vi "BBO_Spare.vi"(9 "카메라 X":dbl=12.0, 11 "클러스터":T2={{"정지할 차이값"=0.08, "흰색과 밖 차이값"=0.15, "흰/검 반 값 "=0.3}, {"4: 오른각도"=122.0, "4: 뒷쪽각도"=0.0, "5: 오른각도"=120.0, "5: 앞쪽각도"=245.0, "6: 왼쪽각도"=245.0, "6: 앞쪽각도"=120.0}, {"2: 공각도"=233.0, "2: 굴릴각도"=60.0}}) -> (3 "ROI":T1={"Global Rectangle"=[536, 448, 795, 574], "Contours"=[{"Contour Type"=0, "ROI Type"=3, "Points"=[536, 448, 795, 574]}]})   [LabVIEW 2014]
doc: "The myRIO Project template acquires acceleration data from the onboard accelerometer and displays the changes of acceleration values in a waveform chart."
uses:
  <vilib>/userdefined/High Color/IMAQdx.ctl
  <vilib>/vision/driver/NI_Vision_Acquisition_Software.lvlib
  <vilib>/vision/NI_Vision_Development_Module.lvlib
panel:
  out "시간체크":u32=8202
  in  "Range":cluster{"Lower value":sgl, "Upper value":sgl}={"Lower value"=128.0, "Upper value"=255.0} {"Upper value" format="%.2f"; "Lower value" format="%.2f"}
  in  "조정":dbl=300.0
  in  "수평(뒤로) 초":u32=150
  out "Number of Particles":i32=4
  in  "Local":T3={"Object Type"=0, "Method"=1, "Niblack Deviation Factor"=1.0, "Window"={"Width"=20, "Height"=20}} {"Niblack Deviation Factor" min=0.0 max=1.0 format="%.2f"; "Method" items=["Niblack", "Background Correction"]; "Object Type" items=["Bright Objects", "Dark Objects"]}
  out "숫자형 컨트롤":i32=8
  in  "Select Servo 2":string(combo)="Servo 2"
  out "볼링핀을찾았는가":bool=TRUE
  in  "공 굴릴 범위":dbl=5.0
  in  "작게 움직이는 범위":dbl=500.0
  in  "좌우모터":i16=25
  out "Image 2":T4(plugin-control)
  out "Image":T4(plugin-control)
  # "Control Motor"
  # "Read Encoder"
  # "중간 22"
  # "25"
  # "1,3핀 12"
  # "1일때 + 0일때 -"
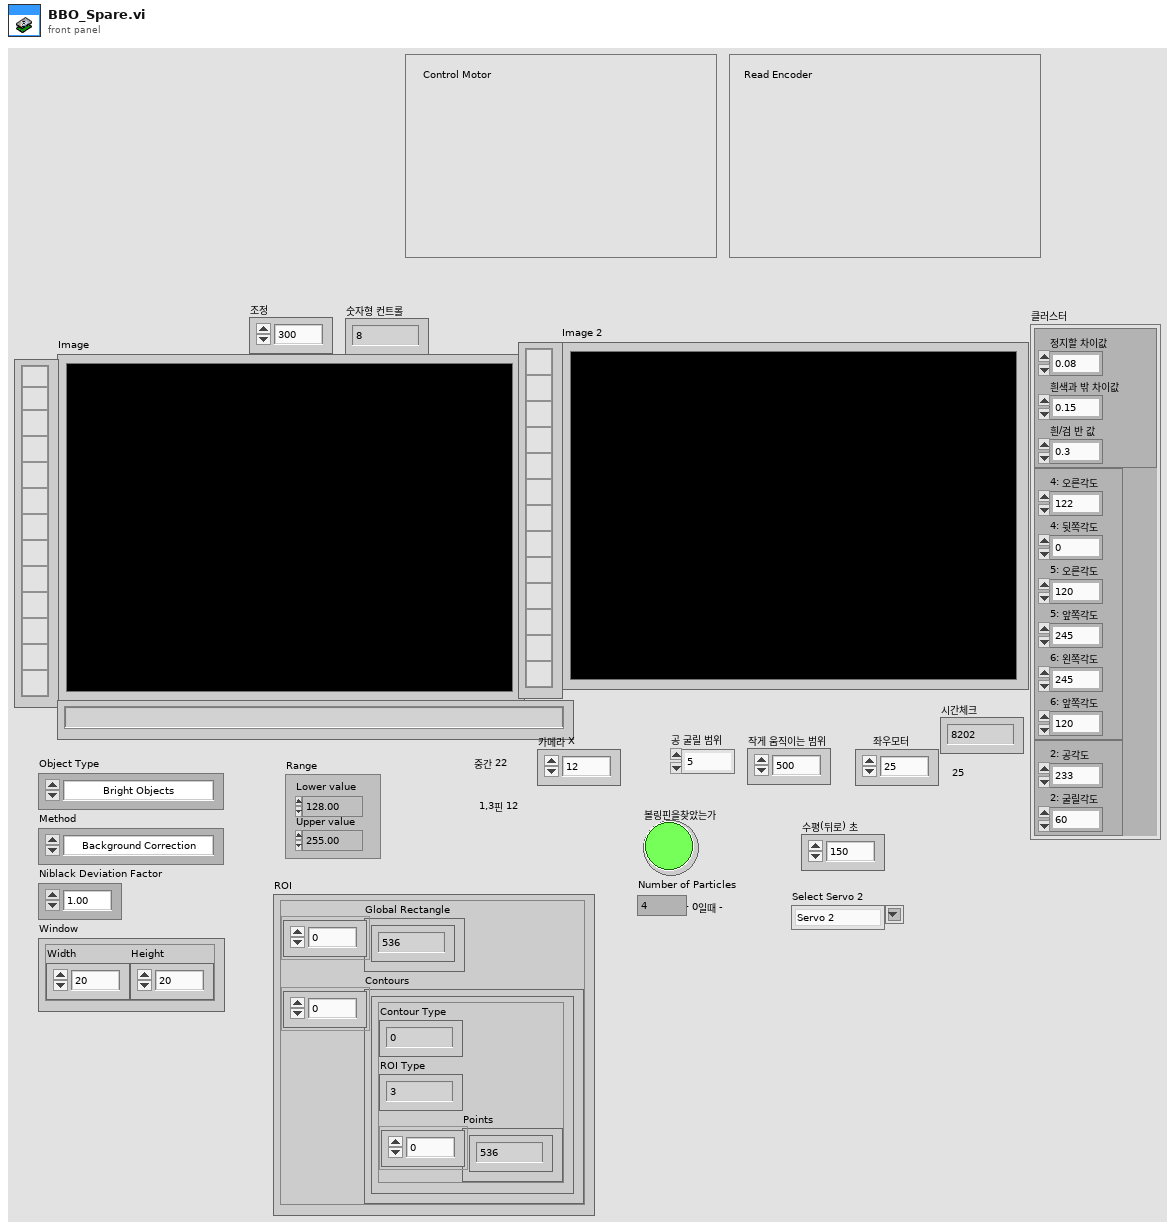
[diagram p1: front panel]
types:
  T1 = cluster{"Global Rectangle":i32[], "Contours":cluster{"Contour Type":u32, "ROI Type":u32, "Points":i32[]}[]}
  T2 = cluster{cluster{"정지할 차이값":dbl, "흰색과 밖 차이값":dbl, "흰/검 반 값 ":dbl}, cluster{"4: 오른각도":dbl, "4: 뒷쪽각도":dbl, "5: 오른각도":dbl, "5: 앞쪽각도":dbl, "6: 왼쪽각도":dbl, "6: 앞쪽각도":dbl}, cluster{"2: 공각도":dbl, "2: 굴릴각도":dbl}}
  T3 = cluster{"Object Type":u32, "Method":u32, "Niblack Deviation Factor":dbl, "Window":cluster{"Width":i32, "Height":i32}}
  T4 = typedef "IMAQ Image.ctl" = refnum<image>
  T5 = typedef "IMAQdx.ctl" = refnum<k21>
  T6 = typedef "IMAQ Rectangle" = cluster{"Left":i32, "Top":i32, "Right":i32, "Bottom":i32, "Rotation":dbl}
  T7 = cluster{"Niblack Deviation Factor":dbl, "Niblack Deviation Factor":dbl}
  T8 = typedef "Image Type" = u32
  T9 = cluster{"Area":dbl, "Number of Holes":dbl, "Bounding Rect":cluster{"Left":dbl, "Top":dbl, "Right":dbl, "Bottom":dbl}, "Center of Mass":cluster{"X":dbl, "Y":dbl}, "Orientation":dbl, "Dimensions":cluster{"Width":dbl, "Height":dbl}}[]
  T10 = cluster{"Left":dbl, "Top":dbl, "Right":dbl, "Bottom":dbl}
  T11 = typedef "ROI Descriptor" = cluster{"Global Rectangle":i32[], "Contours":cluster{"ID":enum32{"External", "Internal"}, "Type":u32, "Coordinates":i32[]}[]}
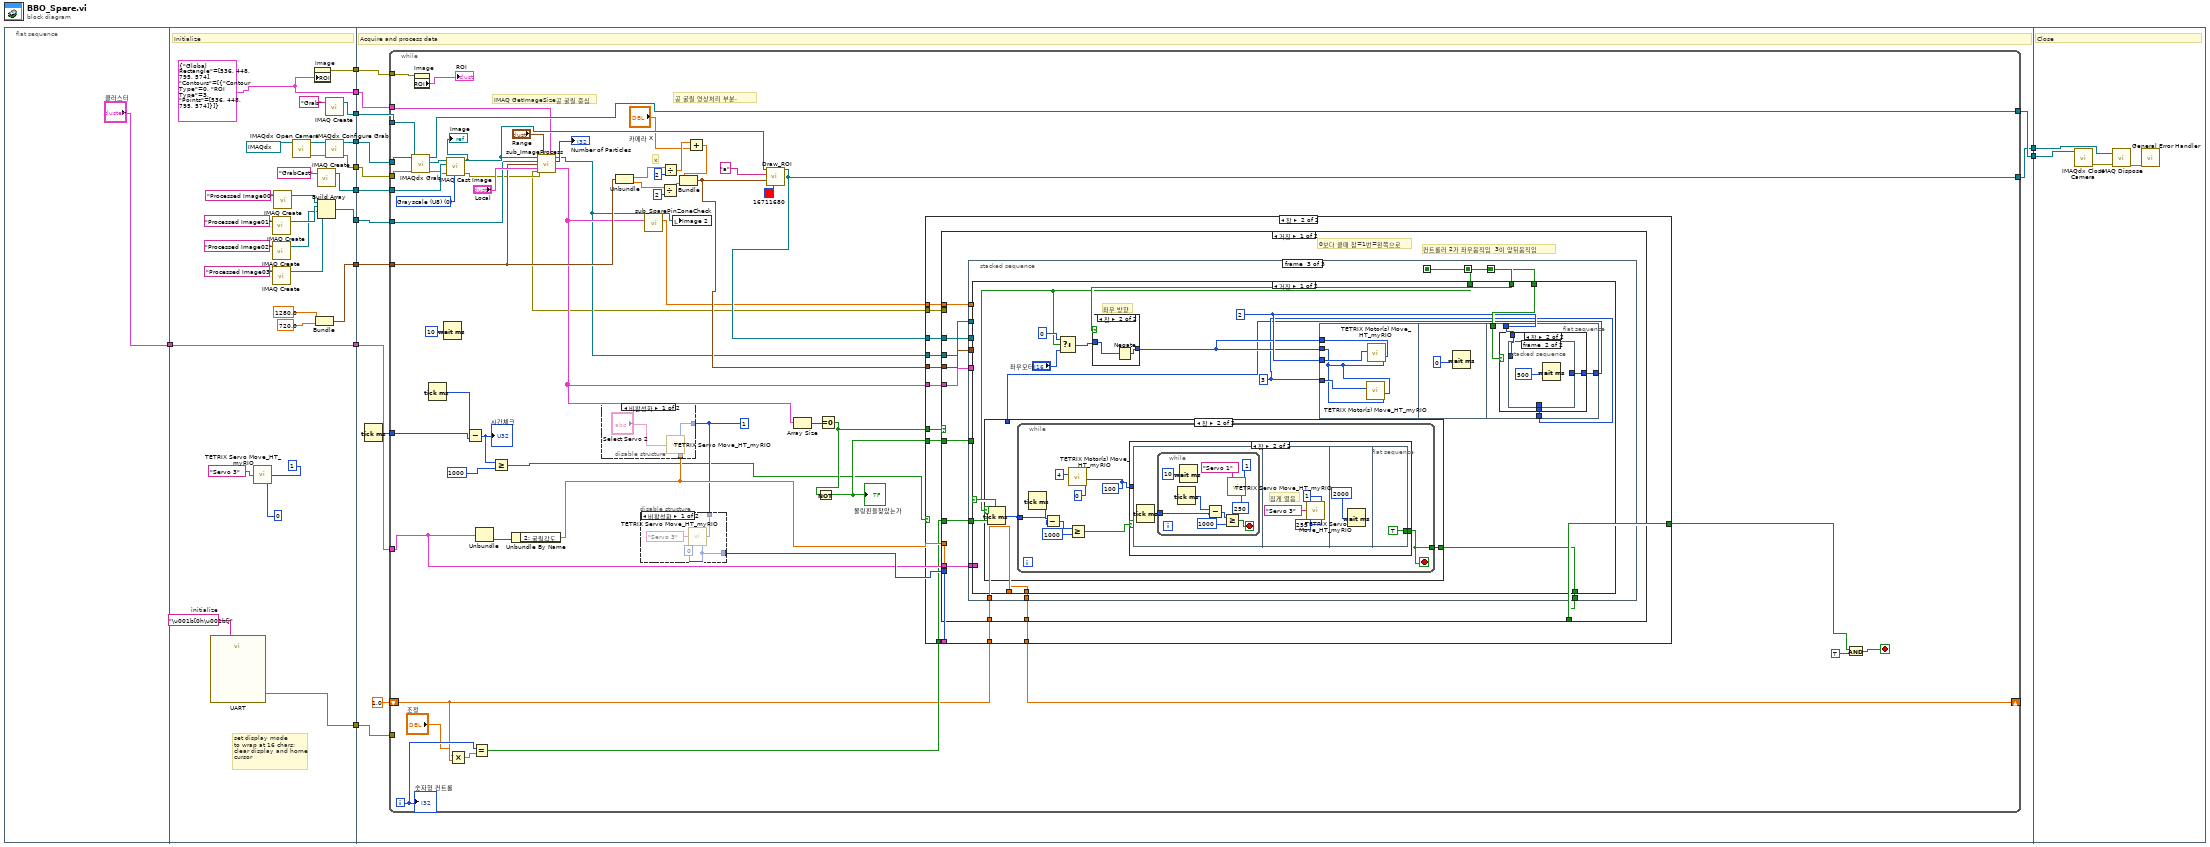
[diagram p0: block diagram]
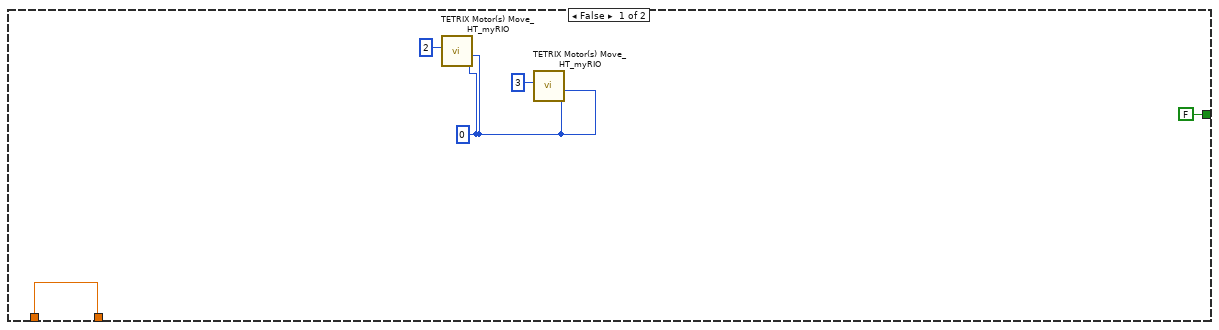
[diagram p4: hidden frame]
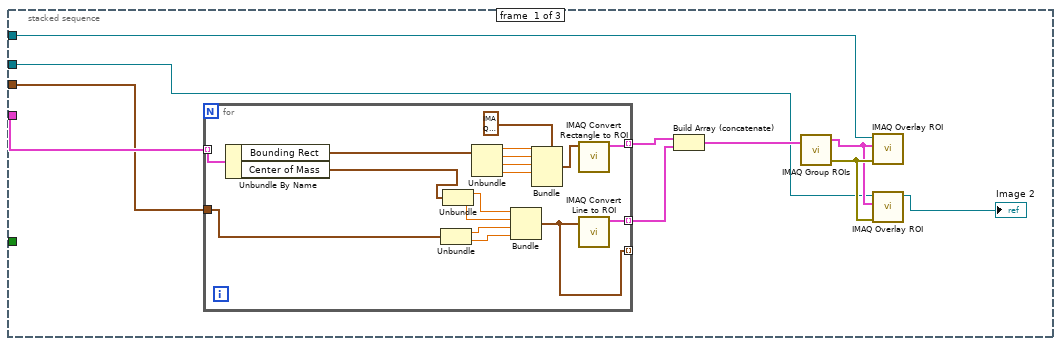
[diagram p5: hidden frame]
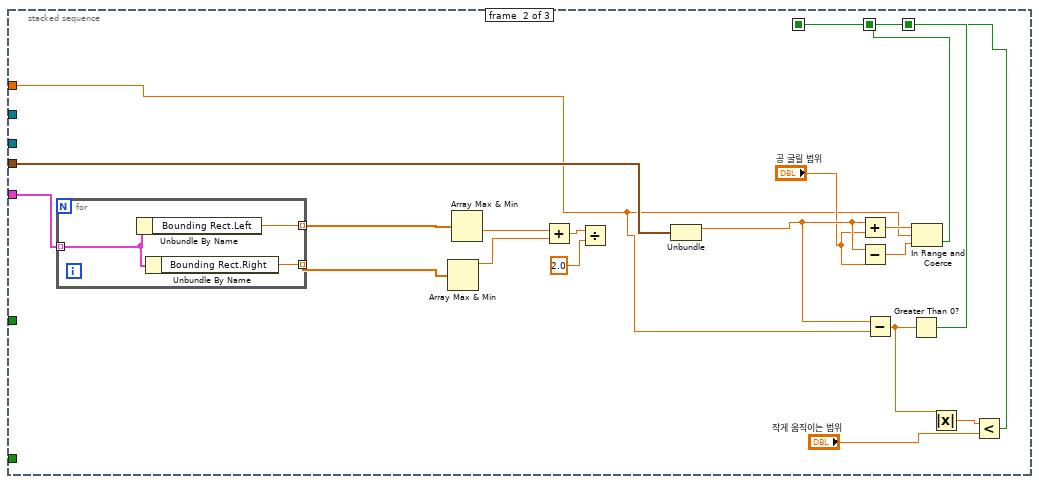
[diagram p6: hidden frame]
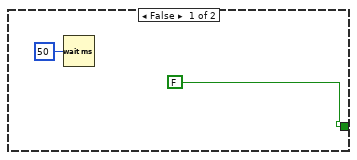
[diagram p7: hidden frame]
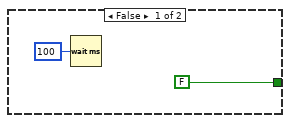
[diagram p8: hidden frame]
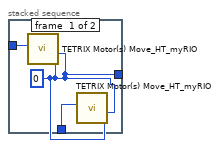
[diagram p10: hidden frame]
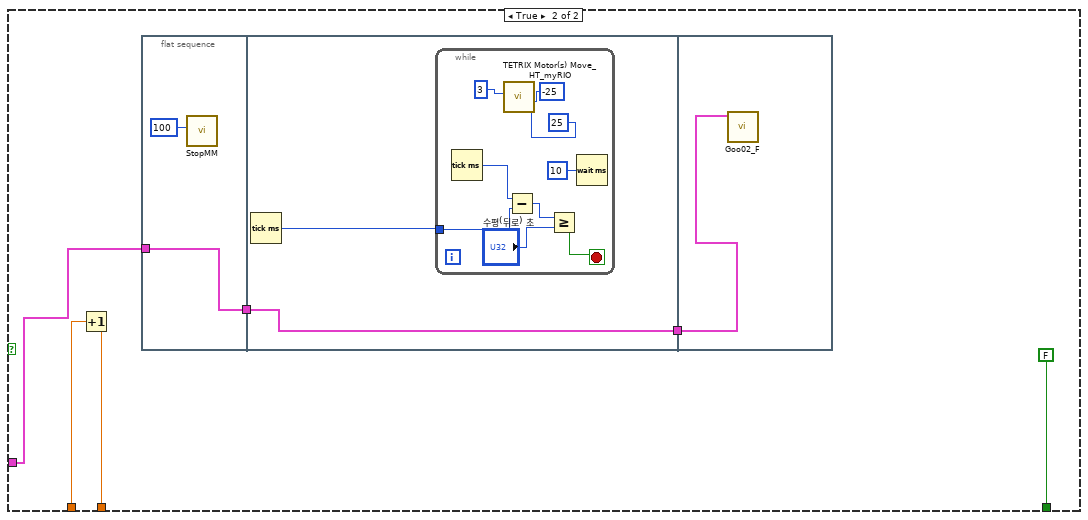
[diagram p12: hidden frame]
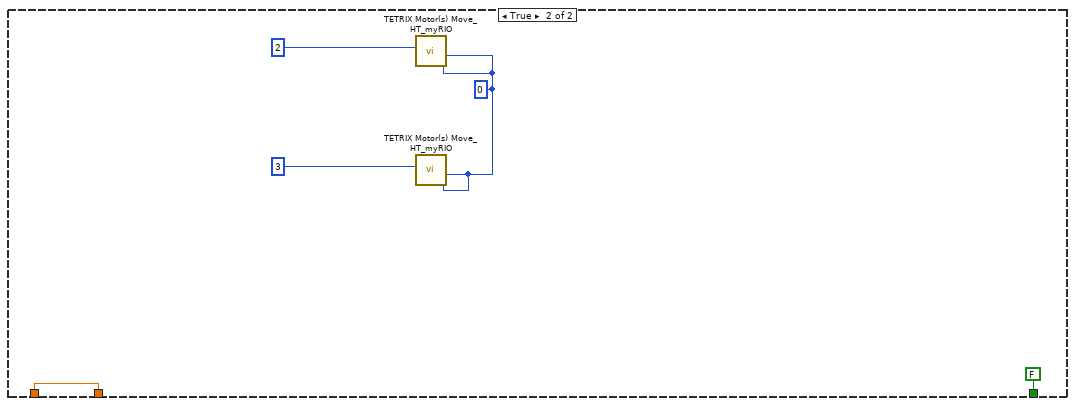
[diagram p13: hidden frame]
diagram:
  n1 = flat-sequence {
    tunnel: ["클러스터"] -> w3
    tunnel: [w40] -> w13
    tunnel: [w39] -> w12
    tunnel: [w38] -> w11
    tunnel: [w26] -> w10
    tunnel: [w36] -> w9
    tunnel: [w33] -> w6
    tunnel: [w30] -> w5
    tunnel: [w21] -> w4
    tunnel: w3 -> [w21]
    tunnel: [w15] -> w2
    tunnel: [w19] -> w1
    tunnel: w13 -> [w57]
    tunnel: w12 -> [w56]
    tunnel: w11 -> [w55]
    tunnel: [w52] -> w8
    tunnel: [w54] -> w7
    tunnel: w10 -> [w53]
    tunnel: w9 -> [w51]
    tunnel: w6 -> [w50]
    tunnel: w5 -> [w49]
    tunnel: w4 -> [w47]
    tunnel: w2 -> [w45]
    tunnel: w1 -> [w46]
    tunnel: w8 -> [w298]
    tunnel: w7 -> [w297]
    frame #0 {
    }
    frame #1 {
      w15 = T1 {"Global Rectangle"=[536, 448, 795, 574], "Contours"=[{"Contour Type"=0, "ROI Type"=3, "Points"=[536, 448, 795, 574]}]} ("ROI")
      w35 = "\u001b[0h\u001b[j"  # initialize
      # "set display mode\nto wrap at 16 chars;\nclear display and home\ncursor"
      # "Initialize"
      n2 = call "UART"("Characters to Write"=w35) -> ("error out"=w36:errorcluster)  [unwired: 25 in, 1 out]
      n3 = call <vilib>:"TETRIX Servo Move_HT_myRIO.vi"("Servo Position (0 - 255)"=u8 0, "Controller Daisy Chain Position (1 - 4)"=u8 1, "Select Servo"="Servo 3") -> ()  [unwired: 2 in, 1 out]
      n4 = call "IMAQ Create"("Image Name"="Processed Image01") -> ("New Image"=w27:T4)  [unwired: 3 in, 2 out]
      n5 = call "IMAQ Create"("Image Name"="Processed Image02") -> ("New Image"=w23:T4)  [unwired: 3 in, 2 out]
      n6 = call "IMAQ Create"("Image Name"="Processed Image03") -> ("New Image"=w22:T4)  [unwired: 3 in, 2 out]
      n7 = call "IMAQ Create"("Image Name"="Processed Image00") -> ("New Image"=w28:T4)  [unwired: 3 in, 2 out]
      n8 = call <vilib>:"IMAQdx Open Camera.vi"("Session In"=T5 "cam1") -> ("error out"=w43:errorcluster, "Session Out"=w42:T5)  [unwired: 2 in, 7 out]
      n9 = property on="Image" class="ImageControl"("ROI"=w15) -> (error out=w19:errorcluster)  [unwired: 2 in, 1 out]
      n10 = Bundle("Niblack Deviation Factor"=1280.0, "Niblack Deviation Factor"=720.0) -> (w30:T7)  [unwired: 1 in]
      n11 = call "IMAQ Create"("Image Name"="GrabCast") -> ("New Image"=w33:T4)  [unwired: 3 in, 2 out]
      n12 = Build Array(w28, w27, w23, w22) -> (w26:T4[])
      n13 = call "IMAQ Create"("Image Name"="Grab") -> ("New Image"=w40:T4)  [unwired: 3 in, 2 out]
      n14 = call <vilib>:"IMAQdx Configure Grab.vi"("error in"=w43, "Session In"=w42) -> ("error out"=w38:errorcluster, "Session Out"=w39:T5)  [unwired: 8 out]
    }
    frame #2 {
      # "Acquire and process data"
      n15 = Tick Count (ms)() -> (millisecond timer value=w44:u32)
      n16 = while {
        tunnel: [w112] -> w54
        tunnel: w55 -> [w114]
        tunnel: w56 -> [w115]
        tunnel: w57 -> [w113]
        tunnel: w53 -> [w94]
        tunnel: [w104] -> w52
        tunnel: w51 -> [_]
        tunnel: w50 -> [w99]
        tunnel: w49 -> [w93]
        shift-right: [w85] -> _
        shift-left: 1.0 -> [w83]
        tunnel: w47 -> [w74]
        tunnel: w46 -> [w66]
        tunnel: w45 -> [w65]
        tunnel: w44 -> [w61]
        i -> [w87]
        stop <- w102 stop-if-true
        w73 = T8 0 items=["Grayscale (U8)", "Grayscale (I16)", "Grayscale (SGL)", "Complex (CSG)", "RGB (U32)", "HSL (U32)", "RGB (U64)", "Grayscale (U16)"] ("Image Type")
        w75 = u8 1 ("Controller Daisy Chain Position (1 - 4)")
        # "공 굴릴 영상처리 부분."
        # "IMAQ GetImageSize공 굴릴 중심"
        # "x"
        n17 = call <vilib>:"IMAQdx Grab.vi"("error in"=w114, "Image In"=w113, "Session In"=w115) -> ("error out"=w98:errorcluster, "Image Out"=w100:T4, "Session Out"=w112:T5)  [unwired: 1 in, 5 out]
        n18 = property on="Image" class="ImageControl"(error in=w66) -> ("ROI"=→"ROI":T1)  [unwired: 1 in, 2 out]
        n19 = Tick Count (ms)() -> (millisecond timer value=w62:u32)
        n20 = Wait (ms)(milliseconds to wait=u32 10 ("대기 시간(ms)")) -> ()  [unwired: 1 out]
        n21 = call "IMAQ Cast Image"("Image Type"=w73, "error in (no error)"=w98, "Image Dst"=w99, "Image Src"=w100) -> ("error out"=w72:errorcluster, "Image Dst Out"=w96:T4)  [unwired: 6 in]
        "Image" <- w96
        n22 = Multiply(x="조정", y=w83) -> (x*y=w86:dbl)
        n23 = Subtract(x=w62, y=w61) -> (x-y=w60:u32)
        "시간체크" <- w60
        n24 = Equal?(x=w87, y=w86) -> (x = y?=w84:bool)
        n25 = Unbundle(w74) -> (w77:cluster{"2: 공각도":dbl, "2: 굴릴각도":dbl})  [unwired: 2 out]
        n26 = Greater Or Equal?(x=w60, y=u32 1000) -> (x >= y?=w58:bool)
        n27 = Unbundle By Name(w77) -> ("2: 굴릴각도"=w76:dbl)
        n28 = call "sub_ImageProcess.vi"("참조 번호 입력"=w96, "Range"="Range", "ROI"=w65, "배열"=w94, "클러스터"=w93, "Local"="Local", "에러 입력(에러 없음)"=w72) -> ("참조 번호 출력"=w68:T4, "Number of Particles"=→"Number of Particles":i32, "Particle Reports (Pixels)"=w81:T9, "error out"=w63:errorcluster)  [unwired: 5 in]
        n29 = disable-structure shown="비활성화" {
          disable-tunnel: w76 -> [w120 _]
          disable-tunnel: w75 -> [w119 _]
          frame Disabled {
            n30 = call <vilib>:"TETRIX Servo Move_HT_myRIO.vi"("Servo Position (0 - 255)"=w120, "Controller Daisy Chain Position (1 - 4)"=w119, "Select Servo"="Select Servo 2") -> ()  [unwired: 2 in, 1 out]
          }
          frame Enabled {
          }
        }
        n31 = Unbundle(w93) -> ("Niblack Deviation Factor"=w92:dbl, "Niblack Deviation Factor"=w91:dbl)
        n32 = disable-structure shown="비활성화" {
          disable-tunnel: [w117 _] -> w78
          disable-tunnel: w75 -> [w116 _]
          frame Disabled {
            w117 = u8 0 ("Servo Position (0 - 255)")
            n33 = call <vilib>:"TETRIX Servo Move_HT_myRIO.vi"("Servo Position (0 - 255)"=w117, "Controller Daisy Chain Position (1 - 4)"=w116, "Select Servo"="Servo 3") -> ()  [unwired: 2 in, 1 out]
          }
          frame Enabled {
          }
        }
        n34 = call "sub_SparePinZoneCheck.vi"("Particle Reports (Pixels)"=w81, "참조 번호 입력"=w68) -> ("숫자형"=w79:dbl, "참조 번호 출력"=w80:T4)  [unwired: 8 in]
        n35 = Divide(x=w91, y=2) -> (x/y=w109:dbl)
        n36 = Divide(x=w92, y=2) -> (x/y=w90:dbl)
        n37 = local write "Image 2"(w80) -> ()
        n38 = Add(x=w90, y="카메라 X") -> (x+y=w88:dbl)
        n39 = Bundle(w88, w109) -> (w106:cluster{dbl, dbl})  [unwired: 1 in]
        n40 = call "Draw_ROI.vi"("Color"=u32 16711680, "클러스터"=w106, "Group"="a", "참조 번호 입력"=w96) -> ("참조 번호 출력"=w104:T4)  [unwired: 7 in]
        n41 = Array Size(array=w81) -> (size(s)=w69:i32)
        n42 = Equal To 0?(x=w69) -> (x = 0?=w71:bool)
        n43 = Not(x=w71) -> (.not. x?=w70:bool)
        "볼링핀을찾았는가" <- w70
        n44 = case shown="참" w58 {
          tunnel: w106 -> [_ w141]
          tunnel: w104 -> [_ w140]
          tunnel: [FALSE w139] -> w103
          tunnel: [w123 w138] -> w85
          tunnel: w84 -> [_ w137]
          tunnel: w83 -> [w123 w136]
          tunnel: w81 -> [_ w135]
          tunnel: w79 -> [_ w134]
          tunnel: w78 -> [_ w133]
          tunnel: w76 -> [_ w132]
          tunnel: w74 -> [_ w131]
          tunnel: w71 -> [_ w130]
          tunnel: w70 -> [_ w129]
          tunnel: w68 -> [_ w128]
          tunnel: w63 -> [_ w127]
          frame False {
            w124 = i8 0 ("Motor 1 Power (-100 to 100)\n0 = Stop/Brake\n-128 = Stop/Coast")
            n45 = call <vilib>:"TETRIX Motor(s) Move_HT_myRIO.vi"("Motor 2 Power (-100 to 100)\n0 = Stop/Brake\n-128 = Stop/Coast"=w124, "Motor 1 Power (-100 to 100)\n0 = Stop/Brake\n-128 = Stop/Coast"=w124, "Controller Daisy Chain Position: 1 - 4"=u8 2) -> ()  [unwired: 6 in, 1 out]
            n46 = call <vilib>:"TETRIX Motor(s) Move_HT_myRIO.vi"("Motor 2 Power (-100 to 100)\n0 = Stop/Brake\n-128 = Stop/Coast"=w124, "Motor 1 Power (-100 to 100)\n0 = Stop/Brake\n-128 = Stop/Coast"=w124, "Controller Daisy Chain Position: 1 - 4"=u8 3) -> ()  [unwired: 6 in, 1 out]
          }
          frame True {
            n47 = case shown="거짓" w130 {
              tunnel: w135 -> [w152 _]
              tunnel: w141 -> [w151 _]
              tunnel: w128 -> [w150 _]
              tunnel: w140 -> [w149 _]
              tunnel: [w148 FALSE] -> w139
              tunnel: w127 -> [_ _]
              tunnel: [w147 w292] -> w138
              tunnel: w137 -> [w146 _]
              tunnel: w136 -> [w145 w292]
              tunnel: w134 -> [w144 _]
              tunnel: w132 -> [_ _]
              tunnel: w133 -> [_ _]
              tunnel: w131 -> [w143 _]
              tunnel: w129 -> [w142 _]
              frame False {
                # "0보다 클때 참=1번=왼쪽으로"
                # "컨트롤러 2가 좌우움직임  3이 앞뒤움직임"
                n48 = stacked-sequence {
                  seq-local: [_ w180 _] -> [_ _ w207]
                  seq-local: [_ w187 _] -> [_ _ w209]
                  seq-local: [_ w183 _] -> [_ _ w208]
                  tunnel: w152 -> [w157 w190 _]
                  tunnel: w151 -> [w154 w189 _]
                  tunnel: w150 -> [w156 _ _]
                  tunnel: w149 -> [w155 _ _]
                  tunnel: [_ _ w206] -> w148
                  tunnel: [_ _ w205] -> w147
                  tunnel: w146 -> [_ _ w204]
                  tunnel: w145 -> [_ _ w203]
                  tunnel: w144 -> [_ w181 _]
                  tunnel: w143 -> [_ _ w202]
                  tunnel: w142 -> [_ _ _]
                  frame #0 {
                    n49 = for {
                      tunnel: w157 -> [w179] mode=indexing
                      tunnel: [w171] -> w159 mode=indexing
                      tunnel: w154 -> [w167]
                      tunnel: [w164] -> w161 mode=indexing
                      tunnel: [w163] -> _ mode=indexing
                      n50 = Unbundle By Name(w179) -> ("Bounding Rect"=w177:T10, "Center of Mass"=w170:cluster{"X":dbl, "Y":dbl})
                      n51 = Unbundle(w167) -> (w166:dbl, w165:dbl)
                      n52 = Unbundle(w170) -> ("X"=w169:dbl, "Y"=w168:dbl)
                      n53 = Unbundle(w177) -> ("Left"=w176:dbl, "Top"=w175:dbl, "Right"=w174:dbl, "Bottom"=w173:dbl)
                      n54 = Bundle("X"=w169, "Y"=w168, w166, w165) -> (w163:cluster{"X":dbl, "Y":dbl, dbl, dbl})  [unwired: 1 in]
                      n55 = Bundle(cluster=T6 {"Left"=0, "Top"=0, "Right"=0, "Bottom"=0, "Rotation"=0.0} ("Rectangle"), "Left"=w176, "Top"=w175, "Right"=w174, "Bottom"=w173) -> (w172:T6)  [unwired: 1 in]
                      n56 = call "IMAQ Convert Rectangle to ROI"("Rectangle"=w172) -> ("ROI Descriptor"=w171:T11)  [unwired: 8 in, 1 out]
                      n57 = call "IMAQ Convert Line to ROI"("Line"=w163) -> ("ROI Descriptor"=w164:T11)  [unwired: 8 in, 1 out]
                    }
                    n58 = Build Array (concatenate)(w159, w161) -> (w160:T11[])
                    n59 = call "IMAQ Group ROIs"("ROI Descriptors"=w160) -> ("error out"=w162:errorcluster, "ROI Descriptor out"=w158:T11)  [unwired: 1 in, 2 out]
                    n60 = call "IMAQ Overlay ROI"("error in (no error)"=w162, "ROI Descriptor"=w158, "Image"=w155) -> ()  [unwired: 3 in, 6 out]
                    n61 = call "IMAQ Overlay ROI"("error in (no error)"=w162, "ROI Descriptor"=w158, "Image"=w156) -> ("Image Out"=→"Image 2":T4)  [unwired: 3 in, 5 out]
                  }
                  frame #1 {
                    n62 = for {
                      tunnel: w190 -> [w201] mode=indexing
                      tunnel: [w200] -> w195 mode=indexing
                      tunnel: [w199] -> w197 mode=indexing
                      n63 = Unbundle By Name(w201) -> ("Bounding Rect.Left"=w200:dbl)
                      n64 = Unbundle By Name(w201) -> ("Bounding Rect.Right"=w199:dbl)
                    }
                    n65 = Array Max & Min(array=w197) -> (max value=w198:dbl)  [unwired: 3 out]
                    n66 = Array Max & Min(array=w195) -> (min value=w196:dbl)  [unwired: 3 out]
                    n67 = Add(x=w196, y=w198) -> (x+y=w191:dbl)
                    n68 = Divide(x=w191, y=2.0) -> ()  [unwired: 1 out]
                    n69 = Unbundle(w189) -> (w188:dbl)  [unwired: 1 out]
                    n70 = Add(x=w188, y="공 굴릴 범위") -> (x+y=w193:dbl)
                    n71 = Subtract(x=w188, y="공 굴릴 범위") -> (x-y=w194:dbl)
                    n72 = Subtract(x=w188, y=w181) -> (x-y=w186:dbl)
                    n73 = Greater Than 0?(x=w186) -> (x > 0?=w187:bool)
                    n74 = In Range and Coerce(upper limit=w193, x=w181, lower limit=w194) -> (In Range?=w180:bool)  [unwired: 1 out]
                    n75 = Absolute Value(x=w186) -> (abs(x)=w185:dbl)
                    n76 = Less?(x=w185, y="작게 움직이는 범위") -> (x < y?=w183:bool)
                  }
                  frame #2 {
                    n77 = case shown="거짓" w204 {
                      tunnel: w209 -> [w221 _]
                      tunnel: w208 -> [w220 _]
                      tunnel: w207 -> [w212 _]
                      tunnel: [w210 FALSE] -> w206
                      tunnel: [w215 w276] -> w205
                      tunnel: w203 -> [w215 w275]
                      tunnel: w202 -> [_ w272]
                      frame False {
                        w213 = u8 3 ("Controller 2")
                        w217 = u8 2 ("Controller 2")
                        # "좌우 방향"
                        n78 = case shown="참" w212 {
                          tunnel: w211 -> [_ _]
                          tunnel: [FALSE w224] -> w210
                          frame False {
                            n79 = Wait (ms)(milliseconds to wait=u32 50 ("대기 시간(ms)")) -> ()  [unwired: 1 out]
                          }
                          frame True {
                            n80 = Tick Count (ms)() -> (millisecond timer value=w225:u32)
                            n81 = while {
                              tunnel: w225 -> [w231]
                              tunnel: [w227] -> w224
                              stop <- w227 stop-if-true
                              w226 = i8 100 ("Motor 1 Power (-100 to 100)\n0 = Stop/Brake\n-128 = Stop/Coast")
                              n82 = Tick Count (ms)() -> (millisecond timer value=w232:u32)
                              n83 = Subtract(x=w232, y=w231) -> (x-y=w230:u32)
                              n84 = call <vilib>:"TETRIX Motor(s) Move_HT_myRIO.vi"("Motor 2 Power (-100 to 100)\n0 = Stop/Brake\n-128 = Stop/Coast"=i8 0 ("Motor 2 Power (-100 to 100)\n0 = Stop/Brake\n-128 = Stop/Coast"), "Motor 1 Power (-100 to 100)\n0 = Stop/Brake\n-128 = Stop/Coast"=w226, "Controller Daisy Chain Position: 1 - 4"=u8 4) -> ()  [unwired: 6 in, 1 out]
                              n85 = Greater Or Equal?(x=w230, y=u32 1000) -> (x >= y?=w229:bool)
                              n86 = case shown="참" w229 {
                                tunnel: w226 -> [_ _]
                                tunnel: [FALSE w237] -> w227
                                frame False {
                                n87 = Wait (ms)(milliseconds to wait=u32 100 ("대기 시간(ms)")) -> ()  [unwired: 1 out]
                                }
                                frame True {
                                n88 = flat-sequence {
                                tunnel: [TRUE] -> w237
                                frame #0 {
                                n89 = Tick Count (ms)() -> (millisecond timer value=w238:u32)
                                n90 = while {
                                tunnel: w238 -> [w246]
                                stop <- w244 stop-if-true
                                n91 = Tick Count (ms)() -> (millisecond timer value=w247:u32)
                                n92 = Wait (ms)(milliseconds to wait=u32 10 ("대기 시간(ms)")) -> ()  [unwired: 1 out]
                                n93 = Subtract(x=w247, y=w246) -> (x-y=w245:u32)
                                n94 = Greater Or Equal?(x=w245, y=u32 1000) -> (x >= y?=w244:bool)
                                n95 = call <vilib>:"TETRIX Servo Move_HT_myRIO.vi"("Servo Position (0 - 255)"=u8 250, "Controller Daisy Chain Position (1 - 4)"=u8 1, "Select Servo"="Servo 1") -> ()  [unwired: 2 in, 1 out]
                                }
                                }
                                frame #1 {
                                # "집게 열음"
                                n96 = call <vilib>:"TETRIX Servo Move_HT_myRIO.vi"("Servo Position (0 - 255)"=u8 255, "Controller Daisy Chain Position (1 - 4)"=u8 1, "Select Servo"="Servo 3") -> ()  [unwired: 2 in, 1 out]
                                }
                                frame #2 {
                                n97 = Wait (ms)(milliseconds to wait=u32 2000 ("대기 시간(ms)")) -> ()  [unwired: 1 out]
                                }
                                frame #3 {
                                }
                                }
                                }
                              }
                            }
                          }
                        }
                        n98 = Select(t=i8 0 ("Motor 2 Power (-100 to 100)\n0 = Stop/Brake\n-128 = Stop/Coast"), s=w212, f="좌우모터") -> (s? t:f=w219:i16)
                        n99 = case shown="참" w221 {
                          tunnel: w219 -> [w269 w271]
                          tunnel: [w269 w270] -> w214
                          frame False {
                          }
                          frame True {
                            n100 = Negate(x=w271) -> (-x=w270:i16)
                          }
                        }
                        n101 = flat-sequence {
                          tunnel: w217 -> [w256]
                          tunnel: w214 -> [w255]
                          tunnel: w214 -> [w253]
                          tunnel: w213 -> [w254]
                          tunnel: w217 -> [w261]
                          tunnel: w220 -> [w260]
                          tunnel: [w259] -> w211
                          tunnel: w213 -> [w258]
                          frame #0 {
                            n102 = call <vilib>:"TETRIX Motor(s) Move_HT_myRIO.vi"("Motor 2 Power (-100 to 100)\n0 = Stop/Brake\n-128 = Stop/Coast"=w253, "Motor 1 Power (-100 to 100)\n0 = Stop/Brake\n-128 = Stop/Coast"=w253, "Controller Daisy Chain Position: 1 - 4"=w254) -> ()  [unwired: 6 in, 1 out]
                            n103 = call <vilib>:"TETRIX Motor(s) Move_HT_myRIO.vi"("Motor 2 Power (-100 to 100)\n0 = Stop/Brake\n-128 = Stop/Coast"=w253, "Motor 1 Power (-100 to 100)\n0 = Stop/Brake\n-128 = Stop/Coast"=w255, "Controller Daisy Chain Position: 1 - 4"=w256) -> ()  [unwired: 6 in, 1 out]
                          }
                          frame #1 {
                            n104 = Wait (ms)(milliseconds to wait=u32 0 ("대기 시간(ms)")) -> ()  [unwired: 1 out]
                          }
                          frame #2 {
                            n105 = case shown="참" w260 {
                              tunnel: w261 -> [_ w264]
                              tunnel: [_ w262] -> w259
                              tunnel: w258 -> [_ w263]
                              frame False {
                              }
                              frame True {
                                n106 = stacked-sequence {
                                tunnel: w264 -> [w267 _]
                                tunnel: w263 -> [w266 _]
                                tunnel: [w265 _] -> w262
                                frame #0 {
                                w265 = i8 0 ("Motor 2 Power (-100 to 100)\n0 = Stop/Brake\n-128 = Stop/Coast")
                                n107 = call <vilib>:"TETRIX Motor(s) Move_HT_myRIO.vi"("Motor 2 Power (-100 to 100)\n0 = Stop/Brake\n-128 = Stop/Coast"=w265, "Motor 1 Power (-100 to 100)\n0 = Stop/Brake\n-128 = Stop/Coast"=w265, "Controller Daisy Chain Position: 1 - 4"=w267) -> ()  [unwired: 6 in, 1 out]
                                n108 = call <vilib>:"TETRIX Motor(s) Move_HT_myRIO.vi"("Motor 2 Power (-100 to 100)\n0 = Stop/Brake\n-128 = Stop/Coast"=w265, "Motor 1 Power (-100 to 100)\n0 = Stop/Brake\n-128 = Stop/Coast"=w265, "Controller Daisy Chain Position: 1 - 4"=w266) -> ()  [unwired: 6 in, 1 out]
                                }
                                frame #1 {
                                n109 = Wait (ms)(milliseconds to wait=u32 500 ("대기 시간(ms)")) -> ()  [unwired: 1 out]
                                }
                                }
                              }
                            }
                          }
                        }
                      }
                      frame True {
                        n110 = Increment(x=w275) -> (x+1=w276:dbl)
                        n111 = flat-sequence {
                          tunnel: [w278] -> w273
                          tunnel: w272 -> [w278]
                          tunnel: [w280] -> w274
                          tunnel: w273 -> [w280]
                          tunnel: w274 -> [w291]
                          frame #0 {
                            n112 = call "StopMM.vi"("대기 시간(ms)"=u32 100) -> ()  [unwired: 11 in]
                          }
                          frame #1 {
                            n113 = Tick Count (ms)() -> (millisecond timer value=w281:u32)
                            n114 = while {
                              tunnel: w281 -> [w285]
                              stop <- w283 stop-if-true
                              n115 = Tick Count (ms)() -> (millisecond timer value=w286:u32)
                              n116 = call <vilib>:"TETRIX Motor(s) Move_HT_myRIO.vi"("Motor 2 Power (-100 to 100)\n0 = Stop/Brake\n-128 = Stop/Coast"=i8 25 ("Motor 2 Power (-100 to 100)\n0 = Stop/Brake\n-128 = Stop/Coast"), "Motor 1 Power (-100 to 100)\n0 = Stop/Brake\n-128 = Stop/Coast"=i8 -25 ("Motor 1 Power (-100 to 100)\n0 = Stop/Brake\n-128 = Stop/Coast"), "Controller Daisy Chain Position: 1 - 4"=u8 3) -> ()  [unwired: 6 in, 1 out]
                              n117 = Subtract(x=w286, y=w285) -> (x-y=w284:u32)
                              n118 = Greater Or Equal?(x=w284, y="수평(뒤로) 초") -> (x >= y?=w283:bool)
                              n119 = Wait (ms)(milliseconds to wait=u32 10 ("대기 시간(ms)")) -> ()  [unwired: 1 out]
                            }
                          }
                          frame #2 {
                            n120 = call "Goo02_F.vi"("클러스터"=w291) -> ()  [unwired: 11 in]
                          }
                        }
                      }
                    }
                  }
                }
              }
              frame True {
                w294 = 0
                n121 = call <vilib>:"TETRIX Motor(s) Move_HT_myRIO.vi"("Motor 2 Power (-100 to 100)\n0 = Stop/Brake\n-128 = Stop/Coast"=w294, "Motor 1 Power (-100 to 100)\n0 = Stop/Brake\n-128 = Stop/Coast"=w294, "Controller Daisy Chain Position: 1 - 4"=u8 2) -> ()  [unwired: 6 in, 1 out]
                n122 = call <vilib>:"TETRIX Motor(s) Move_HT_myRIO.vi"("Motor 2 Power (-100 to 100)\n0 = Stop/Brake\n-128 = Stop/Coast"=w294, "Motor 1 Power (-100 to 100)\n0 = Stop/Brake\n-128 = Stop/Coast"=w294, "Controller Daisy Chain Position: 1 - 4"=u8 3) -> ()  [unwired: 6 in, 1 out]
              }
            }
          }
        }
        n123 = And(x=w103, y=TRUE) -> (x .and. y?=w102:bool)
        "숫자형 컨트롤" <- w87
      }
    }
    frame #3 {
      # "Close"
      n124 = call <vilib>:"IMAQdx Close Camera.vi"("Session In"=w297) -> ("error out"=w300:errorcluster)  [unwired: 1 in, 9 out]
      n125 = call "IMAQ Dispose"("Image"=w298, "error in (no error)"=w300) -> ("error out"=w299:errorcluster)  [unwired: 4 in]
      n126 = call <vilib>:"General Error Handler.vi"("error in (no error)"=w299) -> ()  [unwired: 2 in, 13 out]
    }
  }
